vi "Handle Collision.vi"(8 "Cluster":T1, 9 "Column":i32, 10 "Row":i32, 11 "Temp DVR":refnum<data-value>) -> (3 "Temp DVR":refnum<data-value>)   [LabVIEW 2014, in "SquareBattle.lvclass"]
uses:
  SquareBattle.lvclass
  Runner Cluster.ctl
  Runner/Runner.lvclass
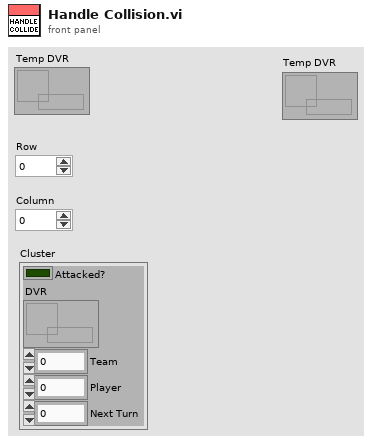
[diagram p1: front panel]
types:
  T1 = typedef "SquareBattle.lvclass/Runner Cluster.ctl" = cluster{"Attacked?":bool, "DVR":refnum<data-value>, "Team":i32, "Player":i32, "Next Turn":i32}
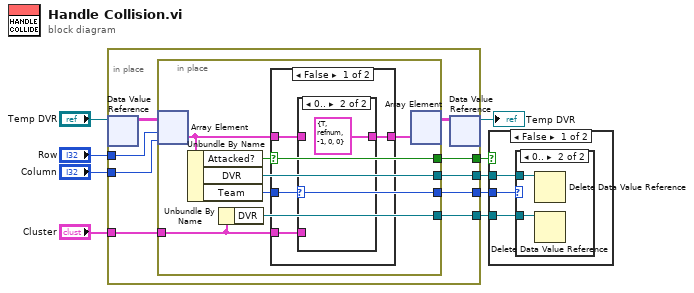
[diagram p0: block diagram]
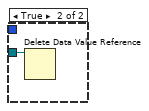
[diagram p3: hidden frame]
diagram:
  n1 = in-place {
    in-place-border: "Row" -> [w17]
    in-place-border: "Column" -> [w16]
    in-place-border: "Cluster" -> [w14]
    in-place-border: [w13] -> w4
    in-place-border: [w12] -> w3
    in-place-border: [w11] -> w2
    in-place-border: [w10] -> w1
    n2 = in-place-dvr #1("Temp DVR") -> (w18:T1[][])  [unwired: 1 out]
    n3 = in-place {
      in-place-border: w14 -> [w23]
      in-place-border: [w22] -> w13
      in-place-border: [w21] -> w12
      in-place-border: [w20] -> w11
      in-place-border: [w19] -> w10
      n4 = in-place-array #2(w18, w17, w16) -> (w24:T1)
      n5 = Unbundle By Name(w24) -> ("Attacked?"=w22:bool, "DVR"=w21:refnum<data-value>, "Team"=w20:i32)
      n6 = Unbundle By Name(w23) -> ("DVR"=w19:refnum<data-value>)
      n7 = case shown="False" w22 {
        tunnel: [w27 w32] -> w25
        tunnel: w24 -> [w28 w32]
        tunnel: w20 -> [w29 _]
        tunnel: w23 -> [w26 _]
        frame False {
          n8 = case shown="0.." w29 {
            tunnel: w28 -> [_ _]
            tunnel: [w30 T1 {"Attacked?"=TRUE, "DVR"=refnum, "Team"=-1, "Player"=0, "Next Turn"=0} ("Cluster")] -> w27
            tunnel: w26 -> [w30 _]
            frame ..-1 {
            }
            frame 0.. {
            }
          }
        }
        frame True {
        }
      }
      n9 = in-place-array #2(w25) -> (w15:T1[][])  [unwired: 2 out]
    }
    n10 = in-place-dvr #1(w15) -> (→"Temp DVR":refnum<data-value>)  [unwired: 1 out]
  }
  n11 = case shown="False" w4 {
    tunnel: w1 -> [w33 w38]
    tunnel: w3 -> [w35 _]
    tunnel: w2 -> [w34 _]
    frame False {
      n12 = case shown="0.." w34 {
        tunnel: w33 -> [_ w37]
        tunnel: w35 -> [_ w36]
        frame ..-1 {
        }
        frame 0.. {
          n13 = Delete Data Value Reference(data value reference=w36) -> ()  [unwired: 1 in, 2 out]
          n14 = Delete Data Value Reference(data value reference=w37) -> ()  [unwired: 1 in, 2 out]
        }
      }
    }
    frame True {
      n15 = Delete Data Value Reference(data value reference=w38) -> ()  [unwired: 1 in, 2 out]
    }
  }
